vi "ROI VI.vi"(1 "index":i32, 2 "Particle Analysis\n(Pixels)":dbl[][](array[numeric]) format="%.2f") -> (0 "ROI":T1)   [LabVIEW 2020]
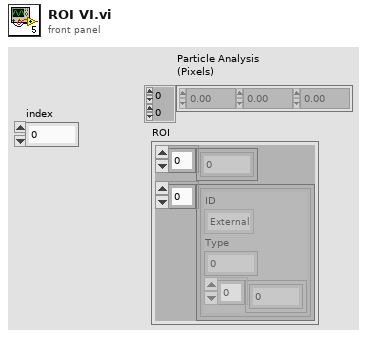
[diagram p1: front panel]
types:
  T1 = cluster{i32[], cluster{"ID":enum32{"External", "Internal"}, "Type":u32, i32[]}[]}
  T2 = cluster{"ID":enum32{"External", "Internal"}, "Type":u32, i32[]}
  T3 = cluster{"ID":enum32{"External", "Internal"}, "Type":u32, i32[]}[]
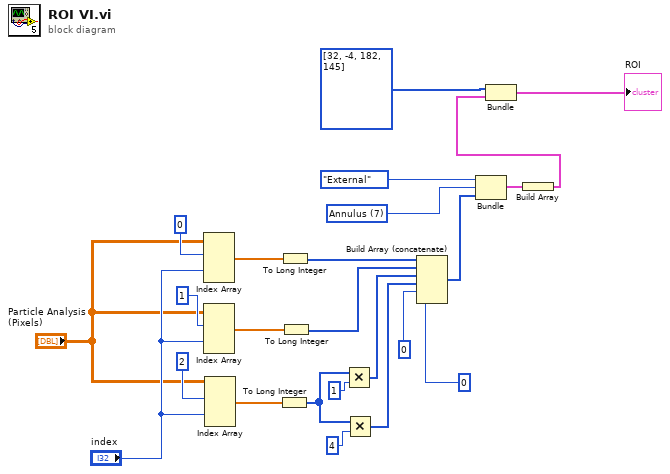
[diagram p0: block diagram]
diagram:
  w13 = u32 7 items=["No Selection", "Point", "Line", "Rectangle", "Oval", "Polygon", "Freehand Region", "Annulus", "Unused2", "Unused3", "Broken Line", "Freehand Line", "Rotated Rectangle"] ("Type")
  n1 = Index Array(array="Particle Analysis\n(Pixels)", index (row) #1=0 ("disabled index (col)"), index (row) #2="index") -> (element #1=w22:dbl[])  [unwired: 2 in, 1 out]
  n2 = Index Array(array="Particle Analysis\n(Pixels)", index (row) #1=1 ("disabled index (col)"), index (row) #2="index") -> (element #1=w23:dbl[])  [unwired: 2 in, 1 out]
  n3 = Index Array(array="Particle Analysis\n(Pixels)", index (row) #1=2 ("disabled index (col)"), index (row) #2="index") -> (element #1=w24:dbl[])  [unwired: 2 in, 1 out]
  n4 = To Long Integer(number=w24) -> (32bit integer=w19:i32[])
  n5 = To Long Integer(number=w22) -> (32bit integer=w21:i32[])
  n6 = To Long Integer(number=w23) -> (32bit integer=w20:i32[])
  n7 = Multiply(x=w19, y=1) -> (x*y=w16:i32[])
  n8 = Multiply(x=w19, y=4) -> (x*y=w15:i32[])
  n9 = Build Array (concatenate)(w21, w20, w16, w15, 0 ("element"), 0 ("element")) -> (w12:i32[])
  n10 = Bundle("ID"=enum32{"External", "Internal"}."External", "Type"=w13, w12) -> (w11:T2)  [unwired: 1 in]
  n11 = Build Array(w11) -> (w2:T3)
  n12 = Bundle(i32[] [32, -4, 182, 145], w2) -> (→"ROI":T1)  [unwired: 1 in]
